vi "Self Test.vi"(8 "error in":errorcluster, 11 "Instruments in":refnum<class "Instruments.lvclass">) -> (0 "error out":errorcluster, 3 "Instruments out":refnum<class "Instruments.lvclass">)   [LabVIEW 2023, in "Instruments.lvlib" / "Instruments.lvclass"]
doc: "This Override VI must be called by ancestor classes\nThis class reads error data and transmits it to the fault handler"
uses:
  Library/Instruments.lvclass
  C:/Users/Public/Documents/Development/builds/Engine/Actor Framework.lvlibp/1abvi3w/vi.lib/ActorFramework/Actor/Actor.lvclass
  builds/Engine/Actor Framework.lvlibp/1abvi3w/vi.lib/ActorFramework/Actor/Read Actor Label.vi
  <vilib>/ErrorRing/Error Ring.xnode
  builds/Engine/Engine.lvlibp/Project/Engine.lvclass
  C:/Users/Public/Documents/Development/builds/Engine/Engine.lvlibp/Project/Engine.lvclass
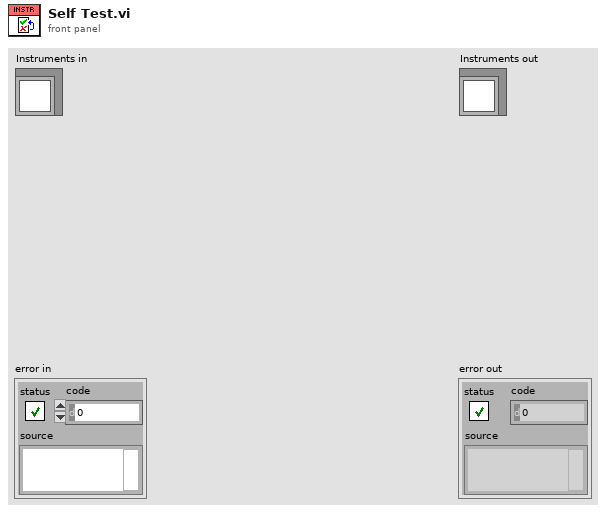
[diagram p1: front panel]
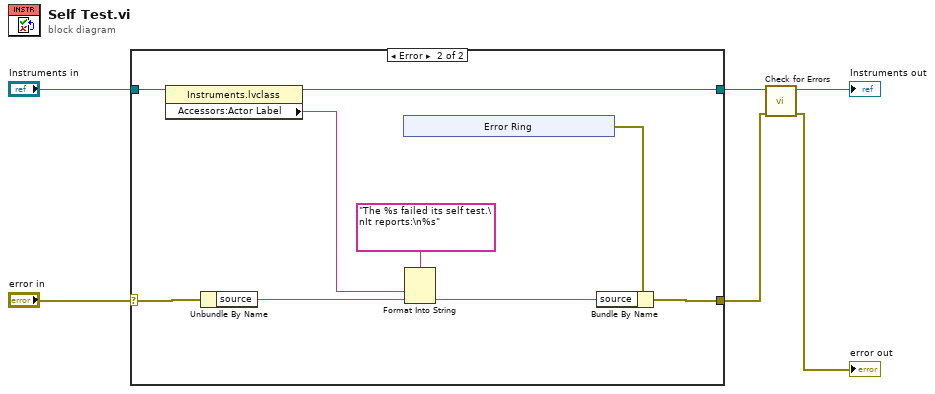
[diagram p0: block diagram]
diagram:
  n1 = case shown="Error" "error in" {
    selector: "error in" -> [w7 w15]
    tunnel: [w7 w16] -> w2
    tunnel: [w8 w13] -> w4
    tunnel: "Instruments in" -> [w8 w14]
    frame No Error {
    }
    frame Error {
      n2 = property class="Instruments.lvclass"(reference=w14) -> (reference out=w13:refnum<class "Instruments.lvclass">, "Accessors:Actor Label"=w10:string)  [unwired: 1 in, 1 out]
      n3 = Unbundle By Name(w15) -> ("source"=w11:string)
      n4 = xnode "Error Ring"() -> ("error out"=w17:errorcluster)
      n5 = Format Into String(format string="The %s failed its self test.\nIt reports:\n%s", w10, w11) -> (resulting string=w9:string)  [unwired: 2 in, 1 out]
      n6 = Bundle By Name(cluster=w17, "source"=w9) -> (w16:errorcluster)
    }
  }
  n7 = call "Check for Errors.vi"("error in"=w2, "Engine in"=w4) -> ("error out"=→"error out":errorcluster, "Engine out"=→"Instruments out":refnum<class "Instruments.lvclass">)  [unwired: 8 in]
